vi "PSDATA_Variant To ArrayDBL.vi"(9 "error in":errorcluster, 10 "Value":variant) -> (1 "error out":errorcluster, 2 "Value":string, 4 "ArrayDBL":dbl[](array[numeric]))   [LabVIEW 2016]
doc: "Developer：YDX"
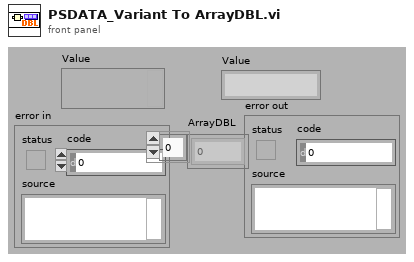
[diagram p1: front panel]
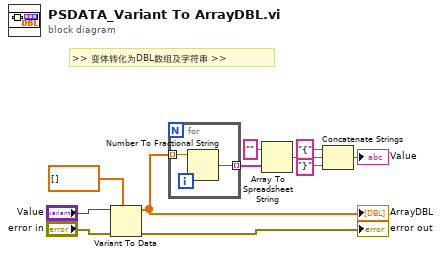
[diagram p0: block diagram]
diagram:
  # ">> 变体转化为DBL数组及字符串 >>"
  n1 = Variant To Data(error in="error in", type=dbl[] [], Variant="Value") -> (data=w7:dbl[], error out=→"error out":errorcluster)
  "ArrayDBL" <- w7
  n2 = for {
    tunnel: [w13] -> w2 mode=indexing
    tunnel: w7 -> [w12] mode=indexing
    n3 = Number To Fractional String(number=w12) -> (F-format string=w13:string)  [unwired: 3 in]
  }
  n4 = Array To Spreadsheet String(array=w2, 3:"" ("format string")) -> (spreadsheet string=w6:string)  [unwired: 1 in]
  n5 = Concatenate Strings("{" ("string"), w6, "}" ("string")) -> (→"Value":string)
